vi "Input_Value_Dialog.vi"(0 "Message to user":string) -> (1 "Value received":dbl format="%.2f", 2 "Ok Out":bool)   [LabVIEW 2011]
uses:
  Controls/ok_button.ctl
  <vilib>/regexp/Match Regular Expression.xnode
panel:
  out "UserMessageDisplay":string
  in  "OK":T1
  in  "Cancel":bool
  in  "Value":dbl format="%.2f"
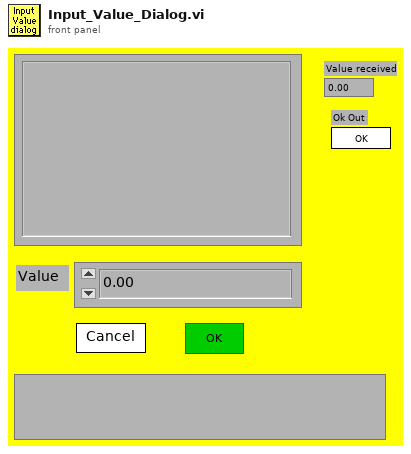
[diagram p1: front panel]
types:
  T1 = typedef "ok_button.ctl" = bool
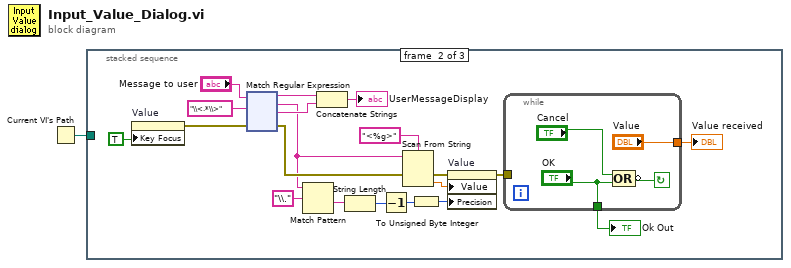
[diagram p0: block diagram]
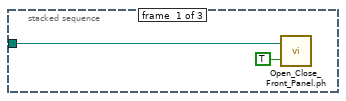
[diagram p2: hidden frame]
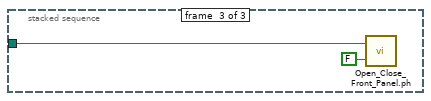
[diagram p3: hidden frame]
diagram:
  n1 = Current VI's Path() -> (path=w1:path)
  n2 = stacked-sequence {
    tunnel: w1 -> [w3 _ w140]
    frame #0 {
      n3 = call "Open_Close_Front_Panel.ph.vi"("Front Panel Window:Open"=TRUE, "VI path"=w3) -> ()  [unwired: 2 out]
    }
    frame #1 {
      n4 = property on="Value" class="DigNum (strict)"("Key Focus"=TRUE) -> (error out=w17:errorcluster)  [unwired: 2 in, 1 out]
      n5 = xnode "Match Regular Expression"("input string"="Message to user", "regular expression"="\\<.*\\>", "error in"=w17) -> ("before match"=w13:string, "whole match"=w10:string, "after match"=w12:string, "error out"=w16:errorcluster)  [unwired: 3 in, 1 out]
      n6 = Match Pattern(string=w10, regular expression="\\.") -> (after substring=w8:string)  [unwired: 1 in, 3 out]
      n7 = Concatenate Strings(w13, w12) -> (→"UserMessageDisplay":string)
      n8 = String Length(string=w8) -> (length=w7:i32)
      n9 = Decrement(x=w7) -> (x-1=w6:i32)
      n10 = Scan From String(format string="<%g>", input string=w10, error in=w16) -> (error out=w15:errorcluster, output 1=w11:dbl)  [unwired: 2 in, 2 out]
      n11 = To Unsigned Byte Integer(number=w6) -> (unsigned 8bit integer=w5:u8)
      n12 = property on="Value" class="DigNum (strict)"(error in=w15, "Value"=w11, "Precision"=w5) -> (error out=w14:errorcluster)  [unwired: 1 in, 1 out]
      n13 = while {
        tunnel: ["OK"] -> w21
        tunnel: ["Value"] -> w23
        tunnel: w14 -> [_]
        stop <- w137 continue-if-true
        n14 = Compound Arithmetic op=OR("Cancel", "OK") -> (invert w137:T1)
      }
      "Value received" <- w23
      "Ok Out" <- w21
    }
    frame #2 {
      n15 = call "Open_Close_Front_Panel.ph.vi"("Front Panel Window:Open"=FALSE, "VI path"=w140) -> ()  [unwired: 2 out]
    }
  }
